vi "RT Array Log.vi"(4 "TimeStamp":dbl format="%#_13g", 6 "def. value":dbl format="%#_13g", 8 "error in":errorcluster, 10 "Array Shift":dbl[](array[numeric]), 11 "Array NW":dbl[](array[numeric])) -> (0 "error out":errorcluster, 1 "def. shift":dbl format="%#_13g", 2 "Array LOG":dbl[](array[numeric]))   [LabVIEW 2017]
doc: "This SubVI used for monitoring change Current TimeStamp\nIf it was change then use other array for output"
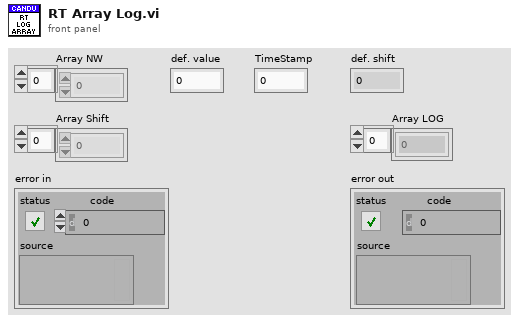
[diagram p1: front panel]
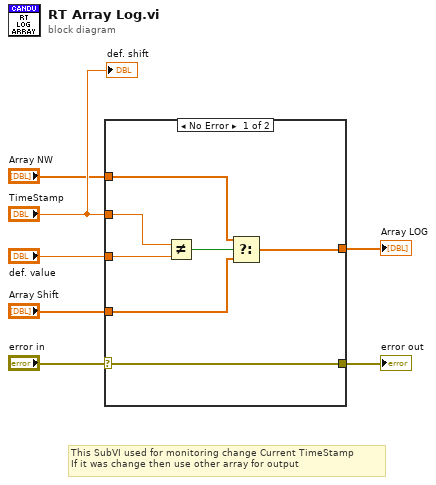
[diagram p0: block diagram]
diagram:
  # "This SubVI used for monitoring change Current TimeStamp\nIf it was change then use other array for output"
  n1 = case shown="No Error" "error in" {
    selector: "error in" -> [w13 w16]
    tunnel: [w13 w16] -> w6
    tunnel: [w12 w15] -> w5
    tunnel: "Array Shift" -> [w11 w15]
    tunnel: "TimeStamp" -> [w10 _]
    tunnel: "def. value" -> [w9 _]
    tunnel: "Array NW" -> [w8 _]
    frame No Error {
      n2 = Not Equal?(x=w10, y=w9) -> (x != y?=w14:bool)
      n3 = Select(t=w8, s=w14, f=w11) -> (s? t:f=w12:dbl[])
    }
    frame Error {
    }
  }
  "error out" <- w6
  "Array LOG" <- w5
  "def. shift" <- "TimeStamp"
